vi "pr_mod_v2.vi"() -> ()   [LabVIEW 2009]
panel:
  out "Numeric":dbl=2.0
  out "Puncte de test":cluster{dbl[], dbl[]}(graph)={[84.94519958704095, 77.87805941285569, 36.46408543048498, 45.84924453380021, 74.3256973936312, 75.91441428356002, 68.82340239567444, 69.55148131924524, 15.127583405957893, 74.04264261594423], [0.5850637660656797, 4.098826936858493, 4.972119784389553, 6.233544547955622, 3.770467965740541, 3.934215834898354, 2.845573429737135, 4.710781221155216, 3.3054868052366397, 2.934253537479086]}
  in  "stop":bool
  out "Presiunea":dbl(slide)=5.116779024612319 scale=0.0..10.0
  in  "Presiune maxima (bar)":dbl(slide)=7.0 scale=0.0..10.0
  out "Temperatura":dbl(slide)=80.43646183515162 scale=0.0..100.0
  in  "Temperatura maxima":dbl(slide)=85.0 scale=0.0..100.0
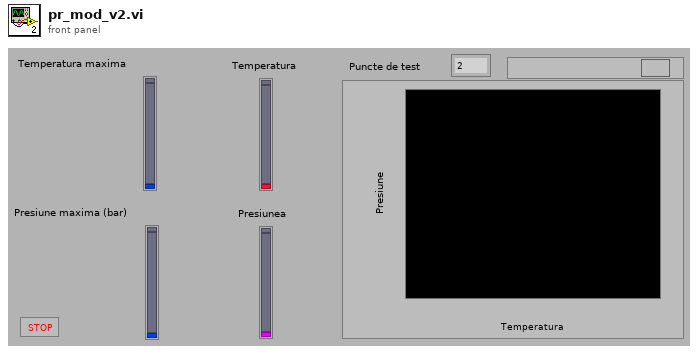
[diagram p1: front panel]
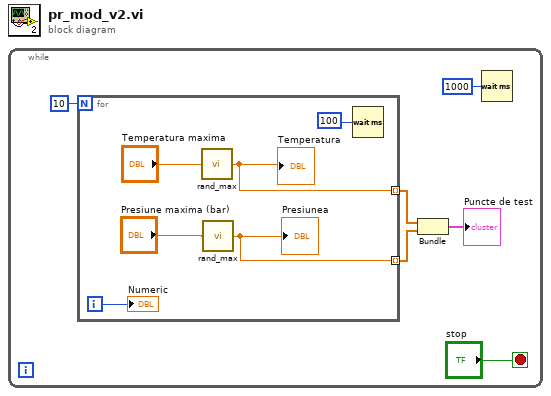
[diagram p0: block diagram]
diagram:
  n1 = while {
    stop <- "stop" stop-if-true
    n2 = for {
      N: 10 -> [_]
      tunnel: [w11] -> w6 mode=indexing
      tunnel: [w10] -> w5 mode=indexing
      i -> [w7]
      n3 = call "rand_max.vi"("Val_max"="Temperatura maxima") -> ("Val_out"=w11:dbl)
      "Temperatura" <- w11
      n4 = call "rand_max.vi"("Val_max"="Presiune maxima (bar)") -> ("Val_out"=w10:dbl)
      "Presiunea" <- w10
      n5 = Wait (ms)(milliseconds to wait=u32 100) -> ()  [unwired: 1 out]
      "Numeric" <- w7
    }
    n6 = Bundle(w6, w5) -> (→"Puncte de test":cluster{dbl[], dbl[]})  [unwired: 1 in]
    n7 = Wait (ms)(milliseconds to wait=u32 1000) -> ()  [unwired: 1 out]
  }
